vi "Get and Set Single Level Detail Coefficients.vi"() -> ()   [LabVIEW 2023]
doc: "This example shows how to read and write the detail coefficients of the discrete wavelet transform result at a certain level.\n\n<b>Instructions:</b>\n1) Run this VI.\n2) Change the value of <b>Wavelet</b> and <b>Level</b>.\n3) Observe the <b>Detail Coefficients at a Level</b>.\n4) Browse the Block Diagram to learn how to read and write the detail coefficients from the result of the WA Discrete Wavelet Transform VI."
uses:
  <vilib>/addons/Wavelet Analysis/typedefs.llb/WA Data.ctl
  <vilib>/addons/Wavelet Analysis/discrete wavelet transform.llb/WA 1D Discrete Wavelet Transform (Array).vi
  <vilib>/addons/Wavelet Analysis/discrete wavelet transform.llb/WA Get Coefficients of 1D Discrete Wavelet Transform (Array).vi
  <vilib>/addons/Wavelet Analysis/discrete wavelet transform.llb/WA Set Coefficients of 1D Discrete Wavelet Transform (Array).vi
  <vilib>/addons/Wavelet Analysis/discrete wavelet transform.llb/WA Inverse 1D Discrete Wavelet Transform (Array).vi
  <vilib>/addons/_Advanced Signal Processing/NI_AdvSigProcWA.lvlib
panel:
  in  "stop":bool
  in  "Level":i32=1 min=1 max=8
  out "Reconstructed Signal":dbl[](graph)
  in  "Wavelet":u16(ring) items=["db02"=0, "db03"=1, "db04"=2, "db05"=3, "db06"=4, "db07"=5, "db08"=6, "db09"=7, "db10"=8, "db11"=9, "db12"=10, "db13"=11, "db14"=12, "Haar"=13, "bior1_3"=14, "bior1_5"=15, "bior2_2"=16, "bior2_4"=17, "bior2_6"=18, "bior2_8"=19, "bior3_1"=20, "bior3_3"=21, "bior3_5"=22, "bior3_7"=23, "bior3_9"=24, "bior4_4 (FBI)"=25, "bior5_5"=38, "bior6_8"=39, "coif1"=26, "coif2"=27, "coif3"=28, "coif4"=29, "coif5"=30, "sym2"=31, "sym3"=32, "sym4"=33, "sym5"=34, "sym6"=35, "sym7"=36, "sym8"=37]
  out "Detail Coefficients at a Level":dbl[](graph)
  out "Signal":dbl[](graph)
  # "Overview: Shows how to read and write the detail coefficients of the discrete wavelet transform result at a certain level.\nRequirements: LabVIEW Full Development System, Advanced Signal Processing Toolkit\nInstructions: \n1. Run this VI.\n2. Change the value of Wavelet and Level.\n3. Observe the Detail Coefficients at a Level.\n4. Browse the block diagram to learn how to read and write the detail coefficients from the result of the WA Discrete Wavelet Transform VI.\n5. Click Stop to stop the VI."
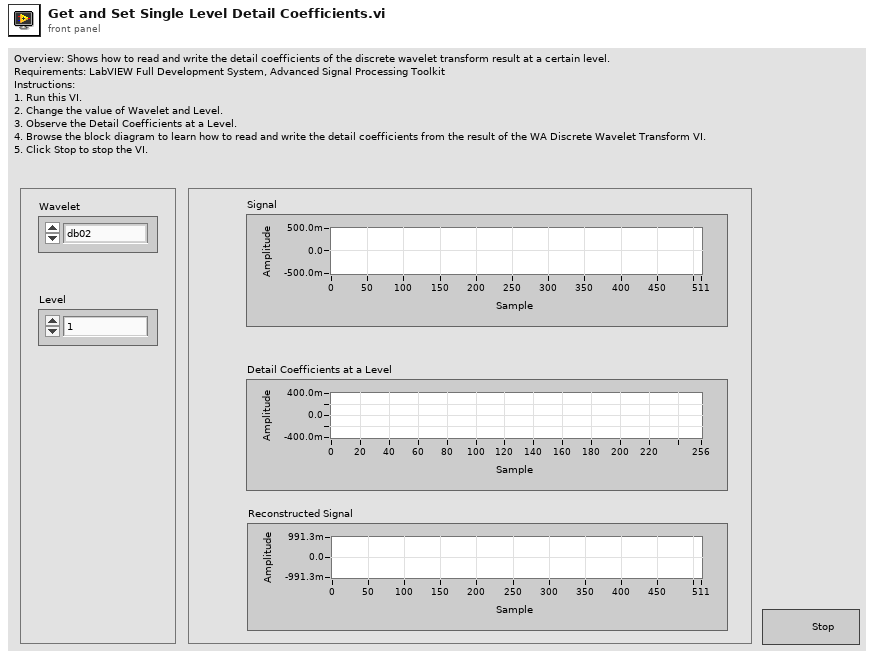
[diagram p1: front panel]
types:
  T1 = typedef "NI_AdvSigProcWA.lvlib/WA Data.ctl" = u16
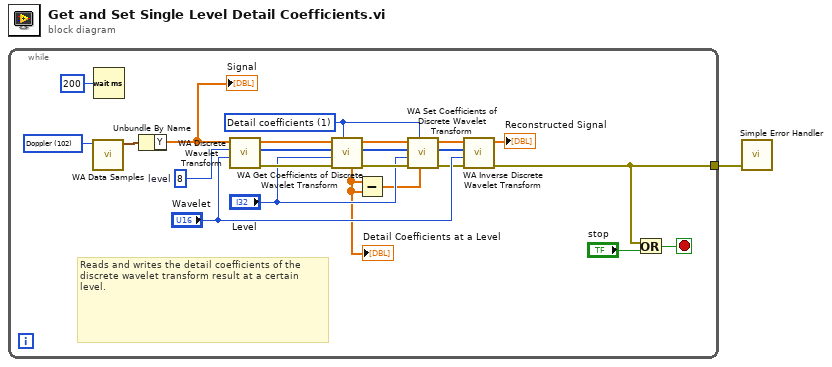
[diagram p0: block diagram]
diagram:
  n1 = while {
    tunnel: [w2] -> w1
    stop <- w18 stop-if-true
    w6 = u16 1 items=["Approximation coefficients", "Detail coefficients"] ("coef type")
    w16 = T1 102 items=["1D Example Data"=100, "-"=101, "Doppler"=102, "HOP"=103, "TF Sine"=104, "Noisy Doppler"=105, "Sea Temperature"=106, "Sp500"=107, "Power Line"=108, "Engine Knocking"=109, "HeaviSine"=110, "Bumps"=111, "Blocks"=112, "Piece Regular"=113, "HypChirps"=114, "LinChirps"=115, "Chirps"=116, "Piece Polynomial"=117, "ECG"=131, "-"=118, "2D Example Data"=119, "-"=120, "Finger Print (Image)"=121, "Iris Flower (Image)"=122, "Mammogram (Image)"=123, "Lake (Image)"=127, "Two Can 1 (Image)"=132, "Two Can 2 (Image)"=133, "Camera Man (Image)"=134] ("data")
    w20 = 8  # level
    # "Reads and writes the detail coefficients of the discrete wavelet transform result at a certain level."
    n2 = call <vilib>:"WA Data Samples.vi"("data"=w16) -> ("signal"=w23:waveform(dbl))  [unwired: 10 out]
    n3 = Wait (ms)(milliseconds to wait=u32 200 ("millisecond multiple")) -> ()  [unwired: 1 out]
    n4 = Unbundle By Name(w23) -> ("Y"=w21:dbl[])
    "Signal" <- w21
    n5 = call-poly <vilib>:"WA Discrete Wavelet Transform.vi"("wavelet"="Wavelet", "levels"=w20, "signal"=w21) -> ("error out"=w13:errorcluster, "length"=w14:i32[], "DWT coef"=w15:dbl[])  [unwired: 1 in, 5 out]
    n6 = call-poly <vilib>:"WA Get Coefficients of Discrete Wavelet Transform.vi"("coef type"=w6, "error in (no error)"=w13, "coef level"="Level", "length"=w14, "DWT coef"=w15) -> ("error out"=w12:errorcluster, "length out"=w10:i32[], "DWT coef out"=w11:dbl[], "selected DWT coef"=w3:dbl[])  [unwired: 3 out]
    "Detail Coefficients at a Level" <- w3
    n7 = Subtract(x=w3, y=w3) -> (x-y=w4:dbl[])
    n8 = call-poly <vilib>:"WA Set Coefficients of Discrete Wavelet Transform.vi"("new DWT coef"=w4, "coef type"=w6, "error in (no error)"=w12, "coef level"="Level", "length"=w10, "DWT coef"=w11) -> ("error out"=w7:errorcluster, "length out"=w8:i32[], "DWT coef out"=w9:dbl[])  [unwired: 3 out]
    n9 = call-poly <vilib>:"WA Inverse Discrete Wavelet Transform.vi"("error in (no error)"=w7, "wavelet"="Wavelet", "length"=w8, "DWT coef"=w9) -> ("error out"=w2:errorcluster, "signal"=→"Reconstructed Signal":dbl[])  [unwired: 6 out]
    n10 = Or(x=w2, y="stop") -> (x .or. y?=w18:bool)
  }
  n11 = call <vilib>:"Simple Error Handler.vi"("error in (no error)"=w1) -> ()  [unwired: 1 in, 8 out]
